vi "Read Frequency.vi"(8 "error in (no error)":errorcluster, 11 "PWM in":refnum<class "LINX-PCA9685 PWM.lvclass">) -> (0 "error out":errorcluster, 2 "Frequency (Hz)":dbl, 3 "PWM out":refnum<class "LINX-PCA9685 PWM.lvclass">)   [LabVIEW 2020, in "LINX-PCA9685 PWM.lvclass"]
uses:
  LINX-PCA9685 PWM.lvclass
  LINX I2C/LINX I2C.lvclass
panel:
  out "Prescaler (raw)":u8
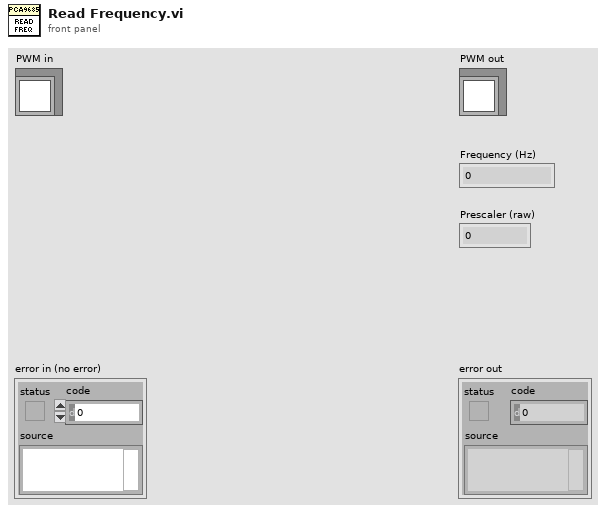
[diagram p1: front panel]
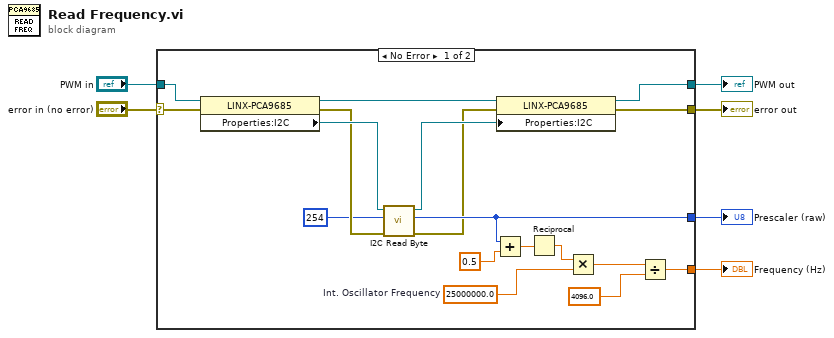
[diagram p0: block diagram]
diagram:
  n1 = case shown="No Error" "error in (no error)" {
    selector: "error in (no error)" -> [w11 w26]
    tunnel: [w8 w26] -> w5
    tunnel: [w14 w25] -> w3
    tunnel: "PWM in" -> [w15 w25]
    tunnel: [w21 _] -> w2
    tunnel: [w17 _] -> w1
    frame No Error {
      w20 = 25000000.0  # Int. Oscillator Frequency
      n2 = property class="LINX-PCA9685"(reference=w15, error in=w11) -> (reference out=w16:refnum<class "LINX-PCA9685 PWM.lvclass">, error out=w10:errorcluster, "Properties:I2C"=w13:refnum<class "LINX I2C.lvclass">)
      n3 = call-dynamic "I2C Read Byte.vi"("error in (no error)"=w10, "Register Address"=u8 254 ("I2C Slave Address 2"), "LINX I2C in"=w13) -> ("error out"=w9:errorcluster, "Byte Read"=w17:u8, "LINX I2C out"=w12:refnum<class "LINX I2C.lvclass">)  [unwired: 6 in]
      n4 = Add(x=w17, y=0.5 ("x")) -> (x+y=w19:dbl)
      n5 = property class="LINX-PCA9685"(reference=w16, error in=w9, "Properties:I2C"=w12) -> (reference out=w14:refnum<class "LINX-PCA9685 PWM.lvclass">, error out=w8:errorcluster)
      n6 = Reciprocal(x=w19) -> (1/x=w18:dbl)
      n7 = Multiply(x=w18, y=w20) -> (x*y=w23:dbl)
      n8 = Divide(x=w23, y=4096.0 ("x")) -> (x/y=w21:dbl)
    }
    frame Error {
    }
  }
  "error out" <- w5
  "PWM out" <- w3
  "Frequency (Hz)" <- w2
  "Prescaler (raw)" <- w1
